vi "Initialize.vi"(8 "error in (no error)":errorcluster, 11 "Arduino Detector in":refnum<class "Arduino Detector.lvclass">) -> (0 "error out":errorcluster, 3 "Arduino Detector out":refnum<class "Arduino Detector.lvclass">)   [LabVIEW 2019, in "Arduino Detector.lvclass"]
uses:
  Arduino Detector.lvclass
  <vilib>/Instr/_visa.llb/VISA Configure Serial Port (Instr).vi
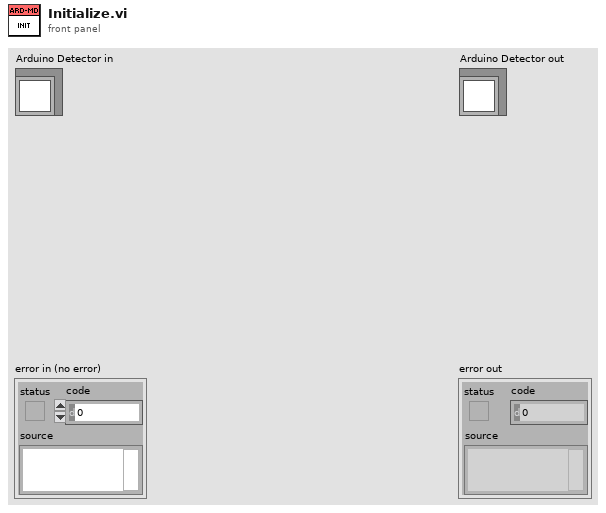
[diagram p1: front panel]
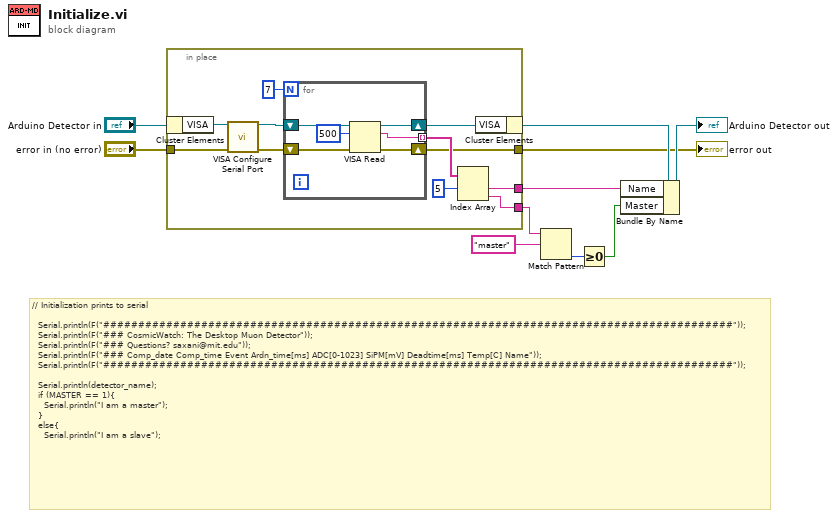
[diagram p0: block diagram]
diagram:
  # "// Initialization prints to serial\n\n  Serial.println(F(\"##########################################################################################\"));\n  Serial.println(F(\"### CosmicWatch: The Desktop Muon Detector\"));\n  Serial.println(F(\"### Questions? saxani@mit.edu\"));\n  Serial.println(F(\"### Comp_date Comp_time Event Ardn_time[ms] ADC[0-1023] SiPM[mV] Deadtime[ms] Temp[C] Name\"));\n  Serial.println(F(\"##########################################################################################\"));\n\n  Serial.println(detector_name);\n  if (MASTER == 1){\n    Serial.println(\"I am a master\");\n  }\n  else{\n    Serial.println(\"I am a slave\");"
  n1 = in-place {
    in-place-border: "error in (no error)" -> [w19]
    in-place-border: [w14] -> w6
    in-place-border: [w12] -> w5
    in-place-border: [w11] -> w4
    n2 = in-place-cluster #1("Arduino Detector in") -> ("VISA"=w20:refnum<visa-resource-name>)
    n3 = call-poly "VISA Configure Serial Port"("VISA resource name"=w20, "error in (no error)"=w19) -> ("VISA resource name out"=w18:refnum<visa-resource-name>, "error out"=w17:errorcluster)  [unwired: 12 in]
    n4 = for {
      N: 7 -> [_]
      shift-right: [w25] -> w16
      shift-left: w18 -> [w27]
      tunnel: [w23] -> w21 mode=indexing
      shift-right: [w22] -> w14
      shift-left: w17 -> [w26]
      n5 = VISA Read(VISA resource name=w27, byte count=u32 500, error in (no error)=w26) -> (VISA resource name out=w25:refnum<visa-resource-name>, read buffer=w23:string, error out=w22:errorcluster)  [unwired: 1 out]
    }
    n6 = Index Array(array=w21, index #1=5 ("index")) -> (element #1=w12:string, element #2=w11:string)  [unwired: 1 in]
    n7 = in-place-cluster #1("VISA"=w16) -> (w8:refnum<class "Arduino Detector.lvclass">)
  }
  "error out" <- w6
  n8 = Match Pattern(string=w4, regular expression="master") -> (offset past match=w2:i32)  [unwired: 1 in, 3 out]
  n9 = Greater Or Equal To 0?(x=w2) -> (x >= 0?=w1:bool)
  n10 = Bundle By Name(cluster=w8, "Name"=w5, "Master"=w1) -> (→"Arduino Detector out":refnum<class "Arduino Detector.lvclass">)
